vi "FHWM.vi"(1 "Input":dbl[](array[numeric])) -> (0 "FWHM":sgl)   [LabVIEW 2011]
uses:
  <vilib>/Analysis/NI_AALBase.lvlib
panel:
  out "Waveform Graph":dbl[](graph)
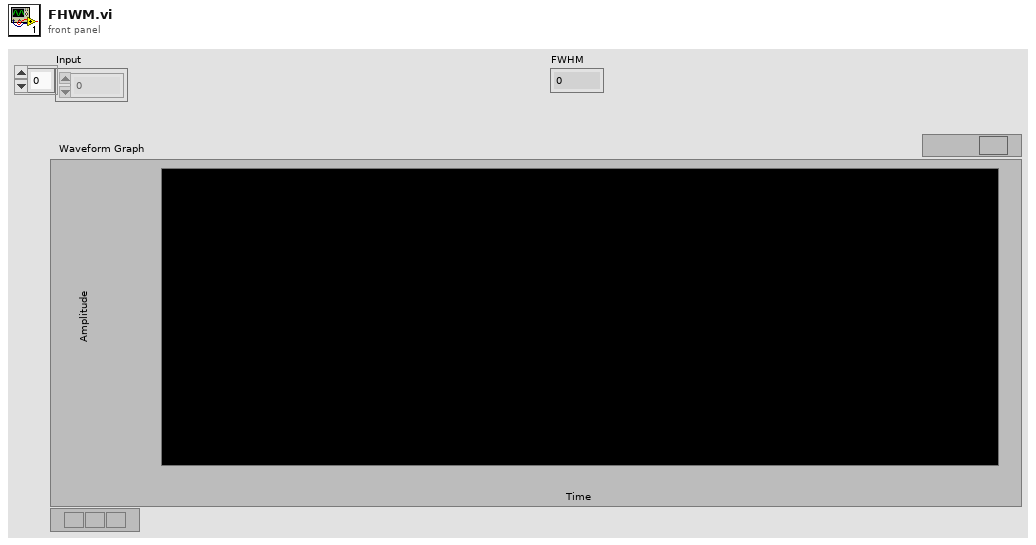
[diagram p1: front panel]
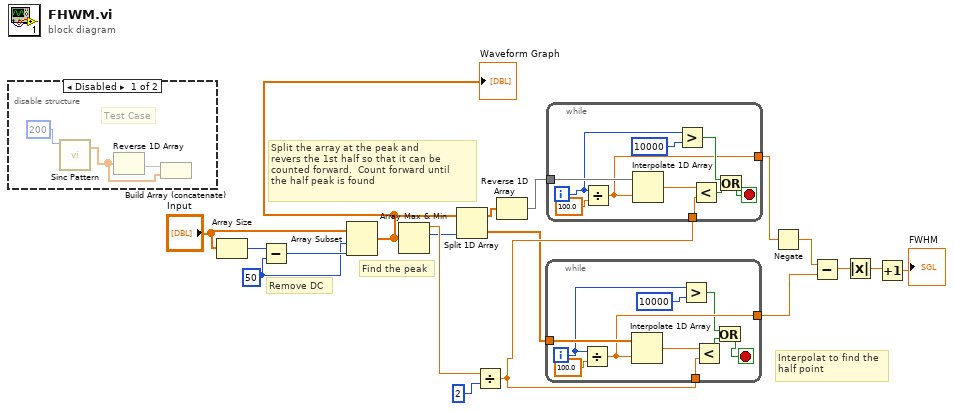
[diagram p0: block diagram]
diagram:
  w16 = 50 ("y")
  # "Interpolat to find the\nhalf point"
  # "Split the array at the peak and\nrevers the 1st half so that it can be \ncounted forward.  Count forward until \nthe half peak is found"
  # "Find the peak"
  # "Remove DC"
  n1 = disable-structure shown="Disabled" {
    frame Disabled {
      # "Test Case"
      n2 = call <vilib>:"Sinc Pattern.vi"("samples"=200) -> ("Sinc Pattern"=w19:dbl[])  [unwired: 3 in, 1 out]
      n3 = Reverse 1D Array(array=w19) -> (reversed array=w20:dbl[])
      n4 = Build Array (concatenate)(w20, w19) -> ()  [unwired: 1 out]
    }
    frame Enabled {
    }
  }
  n5 = Array Size(array="Input") -> (size(s)=w18:i32)
  n6 = Subtract(x=w18, y=w16) -> (x-y=w17:i32)
  n7 = Array Subset(array="Input", index=w16, length=w17) -> (w4:dbl[])
  "Waveform Graph" <- w4
  n8 = Array Max & Min(array=w4) -> (max value=w11:dbl, max index (indices)=w3:i32)  [unwired: 2 out]
  n9 = Split 1D Array(array=w4, index=w3) -> (first subarray=w8:dbl[], second subarray=w6:dbl[])
  n10 = Divide(x=w11, y=2) -> (x/y=w7:dbl)
  n11 = Reverse 1D Array(array=w8) -> (reversed array=w5:dbl[])
  n12 = while {
    tunnel: w6 -> [w31]
    tunnel: [w28] -> w12
    tunnel: w7 -> [w27]
    i -> [w22]
    stop <- w25 stop-if-true
    n13 = Divide(x=w22, y=sgl 100.0) -> (x/y=w28:sgl)
    n14 = Interpolate 1D Array(1:w28, 2:w31) -> (0:w30:dbl)
    n15 = Greater?(x=w22, y=10000 ("x")) -> (0:w24:bool)
    n16 = Less?(x=w30, y=w27) -> (x < y?=w26:bool)
    n17 = Or(x=w24, y=w26) -> (x .or. y?=w25:bool)
  }
  n18 = while {
    tunnel: w5 -> [w41]
    tunnel: [w34] -> w13
    tunnel: w7 -> [w38]
    i -> [w33]
    stop <- w36 stop-if-true
    n19 = Divide(x=w33, y=sgl 100.0) -> (x/y=w34:sgl)
    n20 = Interpolate 1D Array(1:w34, 2:w41) -> (0:w40:dbl)
    n21 = Greater?(x=w33, y=10000 ("x")) -> (0:w35:bool)
    n22 = Less?(x=w40, y=w38) -> (x < y?=w37:bool)
    n23 = Or(x=w35, y=w37) -> (x .or. y?=w36:bool)
  }
  n24 = Negate(x=w13) -> (-x=w15:sgl)
  n25 = Subtract(x=w15, y=w12) -> (x-y=w14:sgl)
  n26 = Absolute Value(x=w14) -> (abs(x)=w2:sgl)
  n27 = Increment(x=w2) -> (x+1=→"FWHM":sgl)
